vi "Turn_On_LED.vi"(8 "error in (no error)":errorcluster, 10 "State":T1, 11 "Car Wash Indicators":refnum<vi>) -> (0 "error out":errorcluster)   [LabVIEW 2023]
uses:
  Controls/State.ctl
panel:
  out "Debug Tool":bool[](array[boolean])
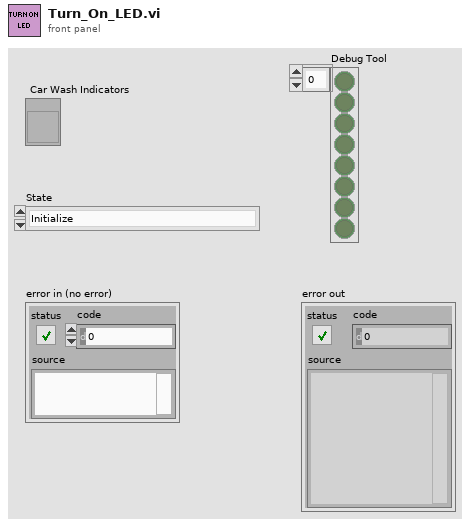
[diagram p1: front panel]
types:
  T1 = typedef "State.ctl" = enum16{"Initialize", "Wait for Something", "Step Completed", "Save Wash Options", "Start Process", "Car Position", "Order Steps to follow", "Underbody Wash", "Bug Remover", "Pre-Soak", "High Pressure Wash", "Low Pressure Wax", "Spot Free Rinse", "Tire Shine Foam", "Air Dry", "Vehicle out of position", "Exit", "Process Complete", "Stop Application"}
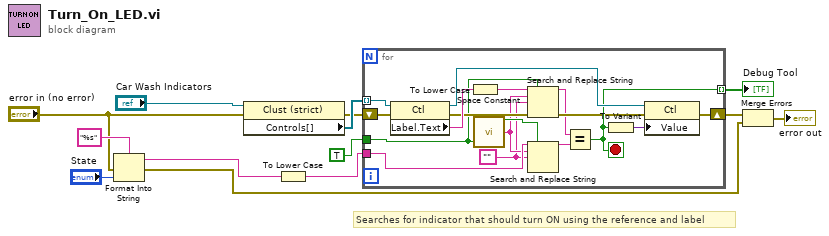
[diagram p0: block diagram]
diagram:
  # "Searches for indicator that should turn ON using the reference and label"
  n1 = Format Into String "Format Into String"(format string="%s", error in="error in (no error)", "State") -> (resulting string=w7:string, error out=w4:errorcluster)  [unwired: 1 in]
  n2 = property class="Clust (strict)"(reference="Car Wash Indicators", error in="error in (no error)") -> (error out=w11:errorcluster, "Controls[]"=w13:refnum<vi>[])  [unwired: 1 out]
  n3 = To Lower Case(string=w7) -> (all lower case string=w2:string)
  n4 = for {
    shift-right: [w27] -> w12
    shift-left: w11 -> [w29]
    tunnel: w13 -> [w28] mode=indexing
    tunnel: w2 -> [w17]
    tunnel: [w24] -> w3 mode=indexing
    tunnel: TRUE ("replace all? (F)") -> [w18]
    stop <- w24 stop-if-true
    w15 = ""
    n5 = property class="Ctl"(reference=w28, error in=w29) -> (reference out=w26:refnum<vi>, error out=w21:errorcluster, "Label.Text"=w23:string)
    n6 = To Lower Case(string=w23) -> (all lower case string=w22:string)
    n7 = call <vilib>:"Space Constant.vi"() -> ("String"=w16:string)
    n8 = Search and Replace String(replace all?=w18, input string=w22, search string=w16, replace string=w15, error in=w21) -> (result string=w19:string, error out=w20:errorcluster)  [unwired: 3 in, 2 out]
    n9 = Search and Replace String(replace all?=w18, input string=w17, search string=w16, replace string=w15) -> (result string=w14:string)  [unwired: 4 in, 3 out]
    n10 = Equal?(x=w19, y=w14) -> (x = y?=w24:bool)
    n11 = To Variant(anything=w24) -> (Variant=w25:variant)
    n12 = property class="Ctl"(reference=w26, error in=w20, "Value"=w25) -> (error out=w27:errorcluster)  [unwired: 1 out]
  }
  "Debug Tool" <- w3
  n13 = Merge Errors(w12, w4) -> (→"error out":errorcluster)
